vi "peak -- rescale back.vi"(5 "norm factor":dbl, 7 "real center":cdb, 10 "scaled point":cdb) -> (2 "real point":cdb)   [LabVIEW 2010]
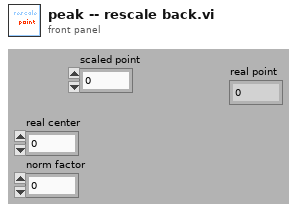
[diagram p1: front panel]
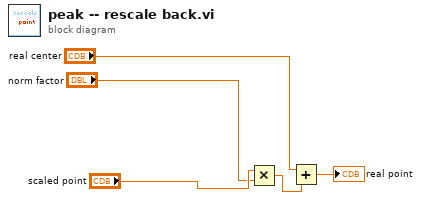
[diagram p0: block diagram]
diagram:
  n1 = Multiply(x="scaled point", y="norm factor") -> (x*y=w3:cdb)
  n2 = Add(x="real center", y=w3) -> (x+y=→"real point":cdb)
